vi "Plot asterisk focus calc.vi"(10 "X-axis?":bool, 11 "Multi-Y?":bool) -> (3 "(*) if focused?":bool)   [LabVIEW 2021, in "RocketPlot.lvlib"]
uses:
  RocketPlot.lvlib
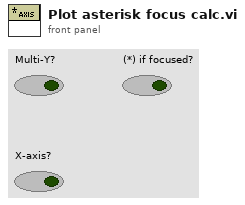
[diagram p1: front panel]
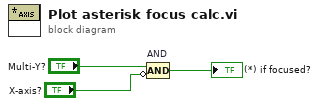
[diagram p0: block diagram]
diagram:
  n1 = Compound Arithmetic op=AND "AND"("Multi-Y?", invert "X-axis?") -> (→"(*) if focused?":bool)
